vi "PID_Timer.vi"() -> ()   [LabVIEW 2013]
panel:
  out "output cluster":cluster{"Slide":dbl, "output":dbl}
  in  "PID gains":T1={"proportional gain (Kc)"=0.8, "integral time (Ti, min)"=0.0001, "derivative time (Td, min)"=1e-05} {"derivative time (Td, min)" format="%.5f"; "integral time (Ti, min)" format="%.5f"; "proportional gain (Kc)" format="%.5f"}
  in  "Slide":dbl(slide)=28.792569659442734 scale=-100.0..100.0
  in  "output range":cluster{"output high":dbl, "output low":dbl}={"output high"=100.0, "output low"=-100.0}
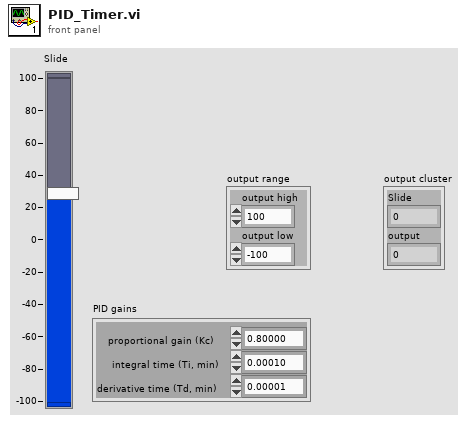
[diagram p1: front panel]
types:
  T1 = cluster{"proportional gain (Kc)":dbl, "integral time (Ti, min)":dbl, "derivative time (Td, min)":dbl}
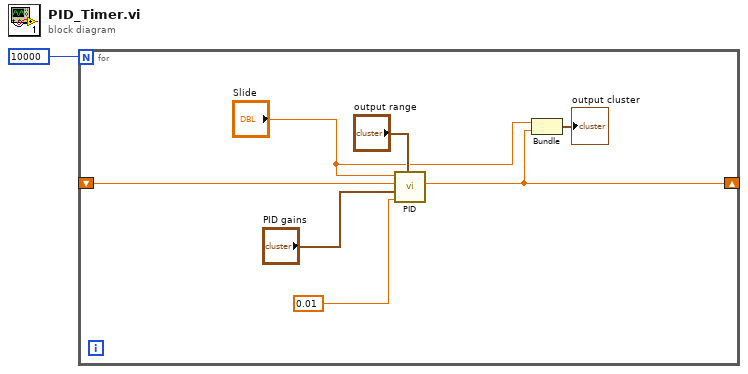
[diagram p0: block diagram]
diagram:
  n1 = for {
    N: 10000 -> [_]
    shift-right: [w4] -> _
    shift-left: _ -> [w2]
    n2 = call "PID.vi"("output range"="output range", "dt (s)"=0.01, "PID gains"="PID gains", "process variable"=w2, "setpoint"="Slide") -> ("output"=w4:dbl)  [unwired: 6 in]
    n3 = Bundle("Slide"="Slide", "output"=w4) -> (→"output cluster":cluster{"Slide":dbl, "output":dbl})  [unwired: 1 in]
  }
